vi "CanSignal.vi"   [LabVIEW 2015]
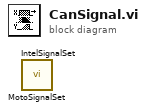
[diagram p0: block diagram]
diagram:
  n1 = call "MotoSignalSet.vi"() -> ()  [unwired: 8 in, 1 out]
  n2 = call "IntelSignalSet.vi"() -> ()  [unwired: 8 in, 1 out]
